vi "Write.vi"(8 "error in (no error)":errorcluster, 10 "write buffer":string, 11 "Serial Logging Decorator In":refnum<class "Serial Logging Decorator.lvclass">) -> (0 "error out":errorcluster, 2 "return count":u32, 3 "Serial Logging Decorator Out":refnum<class "Serial Logging Decorator.lvclass">)   [LabVIEW 2020, in "Serial Logging Decorator.lvclass"]
uses:
  Serial Logging Decorator.lvclass
  Serial Logging Decorator.lvclass/Serial Logging Decorator.ctl
  Log/Log.lvclass
  Serial/Serial.lvclass/Serial.lvclass
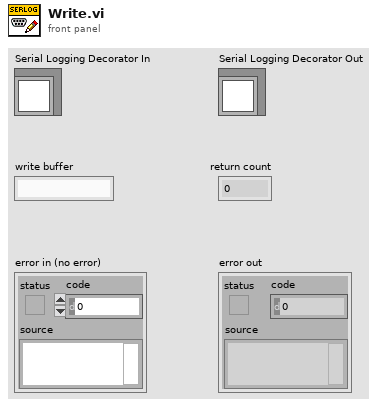
[diagram p1: front panel]
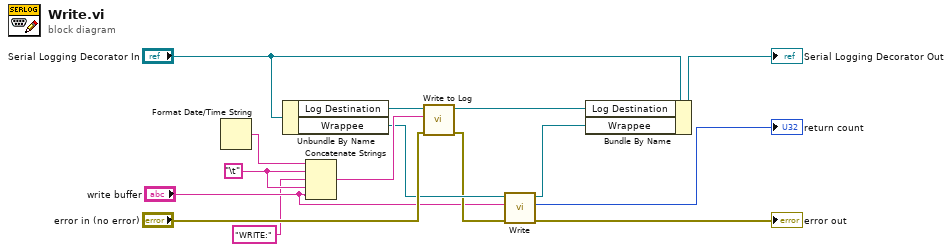
[diagram p0: block diagram]
diagram:
  w2 = "\t" ("string")
  n1 = Format Date/Time String() -> (date/time string=w10:string)  [unwired: 3 in]
  n2 = Unbundle By Name("Serial Logging Decorator In") -> ("Log Destination"=w14:refnum<class "Log.lvclass">, "Wrappee"=w8:refnum<class "Serial.lvclass">)
  n3 = Concatenate Strings(w10, w2, "WRITE:", w2, "write buffer") -> (w9:string)
  n4 = call-dynamic "Write to Log.vi"("error in (no error)"="error in (no error)", "Text to Write"=w9, "Log in"=w14) -> ("error out"=w7:errorcluster, "Log out"=w12:refnum<class "Log.lvclass">)  [unwired: 7 in]
  n5 = call-dynamic "Write.vi"("error in (no error)"=w7, "write buffer"="write buffer", "Serial in"=w8) -> ("error out"=→"error out":errorcluster, "return count"=→"return count":u32, "Serial out"=w5:refnum<class "Serial.lvclass">)  [unwired: 6 in]
  n6 = Bundle By Name(cluster="Serial Logging Decorator In", "Log Destination"=w12, "Wrappee"=w5) -> (→"Serial Logging Decorator Out":refnum<class "Serial Logging Decorator.lvclass">)
